vi "oa_Check dr [OPS] (1 channel).vi"(8 "error in (no error)":errorcluster, 11 "resampled signal":cluster{"r0":dbl, "dr":dbl, "Y":dbl[]} {"r0" format="%.2p"; "dr" format="%.2p"; "Y" format="%.2f"}) -> (0 "error out":errorcluster, 2 "parameter changed":bool, 3 "resampled signal dup":cluster{"r0":dbl, "dr":dbl, "Y":dbl[]} {"r0" format="%.2p"; "dr" format="%.2p"; "Y" format="%.2f"})   [LabVIEW 2017, in "SoundVib_Resampling.lvlib"]
uses:
  <vilib>/addons/Sound and Vibration/Order Analysis/Resample Order Tracking/SoundVib_Resampling.lvlib
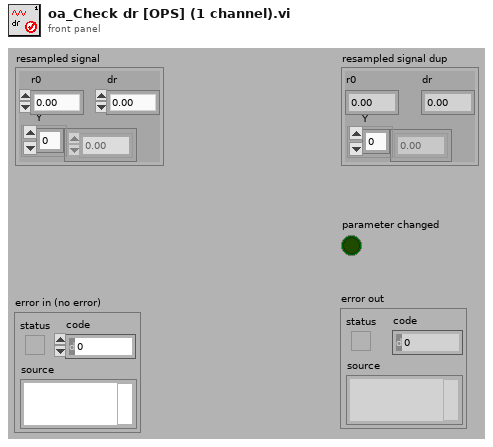
[diagram p1: front panel]
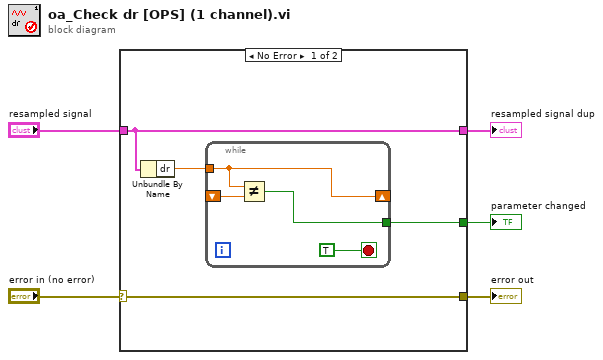
[diagram p0: block diagram]
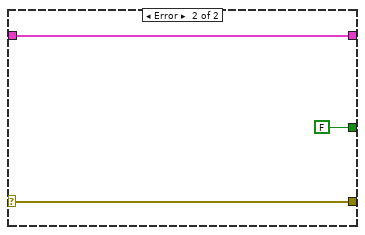
[diagram p2: hidden frame]
diagram:
  n1 = case shown="No Error" "error in (no error)" {
    selector: "error in (no error)" -> [w6 w16]
    tunnel: [w6 w16] -> w4
    tunnel: "resampled signal" -> [w7 w15]
    tunnel: [w8 FALSE] -> w2
    tunnel: [w7 w15] -> w1
    frame No Error {
      n2 = Unbundle By Name(w7) -> ("dr"=w9:dbl)
      n3 = while {
        shift-right: [w12] -> _
        shift-left: _ -> [w13]
        tunnel: w9 -> [w12]
        tunnel: [w10] -> w8
        stop <- TRUE stop-if-true
        n4 = Not Equal?(x=w12, y=w13) -> (x != y?=w10:bool)
      }
    }
    frame Error {
    }
  }
  "resampled signal dup" <- w1
  "error out" <- w4
  "parameter changed" <- w2
